vi "STA - Wave V2 Host.vi"() -> ()   [LabVIEW 2015]
doc: "The continuous acquisition mode tells the FPGA to acquire points indefinitely until a stop command is issued or until an error is encountered (FIFO overflow, module underflow, and so on). \n\nIn this acquisition mode, explicitly call the appropriate rwfm_ConfigTiming VI and set the host application's data buffer to be many times larger than the read size. The examples use a 10X size by default. If the host application's data buffer fills, then the FPGA experiences a FIFO overflow causing the acquisition to stop."
uses:
  <vilib>/rvi/interface/nirviOpenFPGA/nirviOpenFPGA.xnode
  <vilib>/rvi/interface/nirviCloseFPGA/nirviCloseFPGA.xnode
  <vilib>/NI/cRIO Wfm/cRIO Wfm.lvlib
  FPGA Bitfiles/SARAcqMain_9074.lvbitx
  C:/Program Files (x86)/National Instruments/LabVIEW 2015/ProjectTemplates/Source/cRIOWfm/FPGA/[FPGA] SAR Acq Main.vi
  <vilib>/FPGAPlugInAG/Dynamic/niLvFpga_Close_Dynamic.vi
  FPGA Bitfiles/STA-WaveformV0_FPGATarget2_[FPGA]DeltaSigMa_17CDL+fh61Q.lvbitx
  FPGA/[FPGA] DeltaSig Main.vi
  <vilib>/FPGAPlugInAG/cRIO-9112/niLvFpga_Open_cRIO-9112.vi
  <vilib>/rvi/interface/common/dynamic/niFpgaDynamicAddResources.vi
  <vilib>/NI/cRIO Wfm/ChannelConfig.ctl
panel:
  out "Array":timestamp[](array[timestamp])
  out "file path":path
  in  "error in (no error)":errorcluster
  out "error out":errorcluster
  in  "Sample Rate":u32=51200
  in  "stop":bool
  out "Waveform Graph":waveform(sgl)[](graph)
  in  "Channel Info":T1=[{"Channel Name"="Mod1/ai0", "Sensitivity mV_EU"=1000.0, "EU"="V", "dB Ref EU"=1.0}, {"Channel Name"="Mod1/ai1", "Sensitivity mV_EU"=1000.0, "EU"="V", "dB Ref EU"=1.0}, {"Channel Name"="Mod1/ai2", "Sensitivity mV_EU"=1000.0, "EU"="V", "dB Ref EU"=1.0}, {"Channel Name"="Mod1/ai3", "Sensitivity mV_EU"=1000.0, "EU"="V", "dB Ref EU"=1.0}] caption="Channel Name      Scale [mV/EU]        EU           dB Ref [EU]" {"dB Ref EU" format="%#.2p"; "Sensitivity mV_EU" format="%.2f"}
  in  "Samps per Chan":i32=25600 caption="Samples per Channel"
  out "Buffer Backlog":dbl caption="RT Buffer Backlog [%]" format="%#.2g"
  # "Sampling Info"
  # "Channel Info"
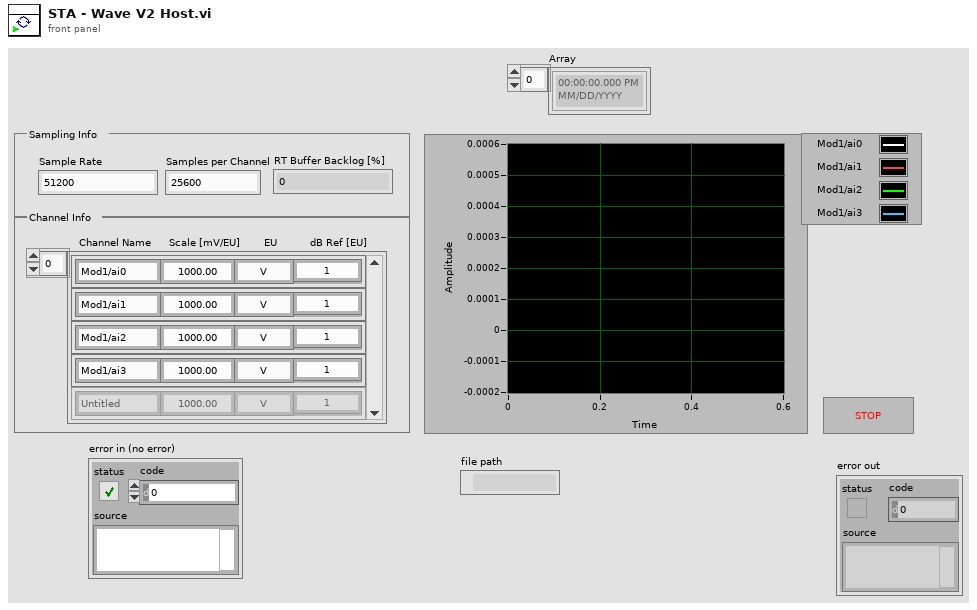
[diagram p1: front panel]
types:
  T1 = typedef "cRIO Wfm.lvlib/ChannelConfig.ctl" = cluster{"Channel Name":string, "Sensitivity mV_EU":dbl, "EU":string, "dB Ref EU":dbl}[]
  T2 = enum16{"open", "open or create", "create or replace", "create", "open (read-only)"}
  T3 = typedef "cRIO Wfm.lvlib/SamplingInfo.ctl" = cluster{"Number of Channels":i32, "Actual Samp Rate":dbl, "Chan Name Array":string[], "EU Chan Array":string[], "dB Ref Chan Array":dbl[]}
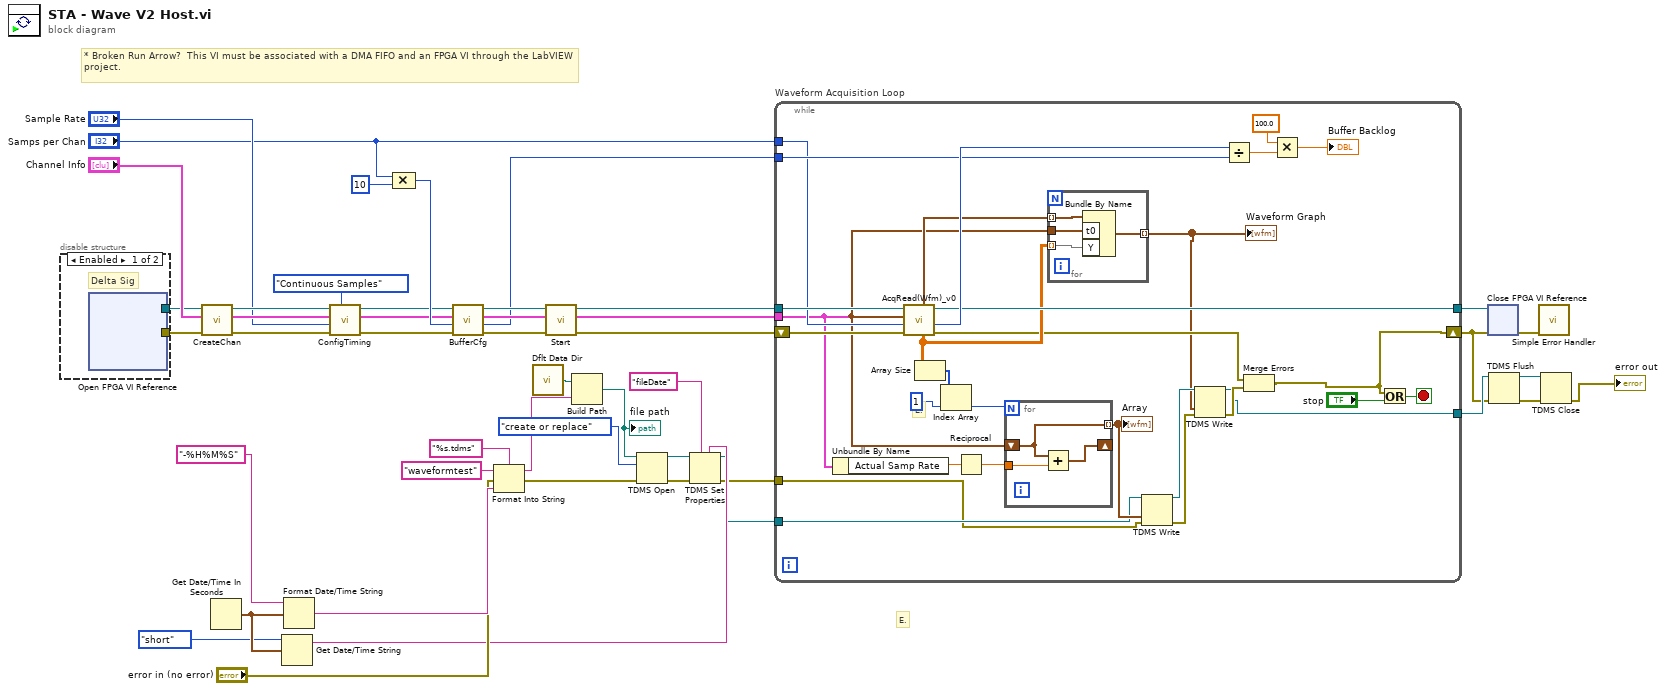
[diagram p0: block diagram]
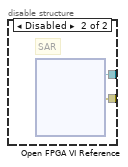
[diagram p2: hidden frame]
diagram:
  # "E."
  # "* Broken Run Arrow?  This VI must be associated with a DMA FIFO and an FPGA VI through the LabVIEW project."
  n1 = disable-structure shown="Enabled" {
    disable-tunnel: [w48 w50] -> w25
    disable-tunnel: [w47 w49] -> w24
    frame Enabled {
      # "Delta Sig"
      n2 = xnode "Open FPGA VI Reference"() -> ("FPGA VI Reference Out"=w48:refnum<k20>, "error out"=w47:errorcluster)  [unwired: 2 in]
    }
    frame Disabled {
      # "SAR"
      n3 = xnode "Open FPGA VI Reference"() -> ("FPGA VI Reference Out"=w50:refnum<k20>, "error out"=w49:errorcluster)  [unwired: 2 in]
    }
  }
  n4 = call <vilib>:"CreateChan.vi"("error in"=w24, "Channel Info"="Channel Info", "Dynamic FPGA Ref"=w25) -> ("error out"=w29:errorcluster, "Sampling Info"=w33:T3, "Dynamic FPGA Ref Out"=w34:refnum<k20>)  [unwired: 1 in, 5 out]
  n5 = Get Date/Time In Seconds() -> (seconds since 1Jan1904=w17:timestamp)
  n6 = Get Date/Time String(date format (0)=enum16{"short", "long", "abbreviated"}."short", seconds (now)=w17) -> (date string=w8:string)  [unwired: 1 in, 1 out]
  n7 = Format Date/Time String(time format string (%c)="-%H%M%S", seconds (now)=w17) -> (date/time string=w19:string)  [unwired: 1 in]
  n8 = call <vilib>:"ConfigTiming.vi"("Sample Mode"=enum16{"Finite Samples", "Continuous Samples"}."Continuous Samples", "error in"=w29, "Sample Rate"="Sample Rate", "Sampling Info In"=w33, "Dynamic FPGA Ref"=w34) -> ("error out"=w30:errorcluster, "Sampling Info Out"=w31:T3, "Dynamic FPGA Ref Out"=w32:refnum<k20>)  [unwired: 3 in, 1 out]
  n9 = Compound Arithmetic op=MULTIPLY("Samps per Chan", 10 ("value")) -> (w39:i32)
  n10 = call <vilib>:"BufferCfg.vi"("error in"=w30, "Buffer Size [Samps per Chan]"=w39, "Sampling Info In"=w31, "Dynamic FPGA Ref"=w32) -> ("error out"=w40:errorcluster, "Buffer Size [Total Samples]"=w36:u32, "Sampling Info Out"=w38:T3, "Dynamic FPGA Ref Out"=w41:refnum<k20>)  [unwired: 4 out]
  n11 = Format Into String(format string="%s.tdms", initial string="waveformtest", error in="error in (no error)", w19) -> (resulting string=w23:string, error out=w6:errorcluster)
  n12 = call <vilib>:"Dflt Data Dir.vi"() -> ("App:Default Data Directory"=w15:path)
  n13 = call <vilib>:"Start.vi"("error in"=w40, "Sampling Info In"=w38, "Dynamic FPGA Ref"=w41) -> ("error out"=w45:errorcluster, "Sampling Info Out"=w37:T3, "Dynamic FPGA Ref Out"=w46:refnum<k20>)  [unwired: 6 out]
  n14 = Build Path(base path=w15, name or relative path=w23) -> (appended path=w11:path)
  "file path" <- w11
  n15 = TDMS Open(8:w6, 10:T2."create or replace" ("operation (0:open)"), 11:w11) -> (0:w14:errorcluster, 3:w13:refnum<k34>)  [unwired: 4 in]
  n16 = TDMS Set Properties(5:w8, 7:"fileDate" ("property names"), 8:w14, 11:w13) -> (0:w4:errorcluster, 3:w5:refnum<k34>)  [unwired: 2 in, 2 out]
  n17 = while "Waveform Acquisition Loop" {
    tunnel: w46 -> [w74]
    tunnel: [w70] -> w44
    tunnel: w37 -> [w66]
    tunnel: w36 -> [w78]
    tunnel: "Samps per Chan" -> [w71]
    shift-right: [w62] -> w2
    shift-left: w45 -> [w80]
    tunnel: w5 -> [w60]
    tunnel: w4 -> [w59]
    tunnel: [w54] -> w3
    stop <- w73 stop-if-true
    # "E."
    n18 = Unbundle By Name(w66) -> ("Actual Samp Rate"=w65:dbl)
    n19 = call <vilib>:"AcqRead(Wfm)_v0.vi"("error in"=w80, "Samps Read per Chan"=w71, "Sampling Info"=w66, "Dynamic FPGA Ref"=w74) -> ("error out"=w63:errorcluster, "Samples Remaining"=w79:u32, "time stamp"=w67:timestamp, "Dynamic FPGA Ref Out"=w70:refnum<k20>, "transposed array"=w68:sgl[][], "Array"=w69:waveform(sgl)[])  [unwired: 2 in]
    n20 = Array Size(array=w68) -> (size(s)=w53:i32[])
    n21 = Index Array(array=w53, index=1) -> (element=w51:i32)
    n22 = Reciprocal(x=w65) -> (1/x=w64:dbl)
    n23 = for {
      N: w51 -> [_]
      shift-right: [w83] -> _
      shift-left: w67 -> [w82]
      tunnel: [w82] -> w61 mode=indexing
      tunnel: w64 -> [w81]
      n24 = Add(x=w82, y=w81) -> (x+y=w83:timestamp)
    }
    "Array" <- w61
    n25 = for {
      tunnel: w69 -> [w87] mode=indexing
      tunnel: w67 -> [w86]
      tunnel: [w85] -> w56 mode=indexing
      tunnel: w68 -> [w84] mode=indexing
      n26 = Bundle By Name(cluster=w87, "t0"=w86, "Y"=w84) -> (w85:waveform(sgl))
    }
    "Waveform Graph" <- w56
    n27 = TDMS Write(0:w60, 9:w61, 11:w59) -> (4:w57:refnum<k34>, 15:w58:errorcluster)  [unwired: 3 in, 2 out]
    n28 = TDMS Write(0:w57, 9:w56, 11:w58) -> (4:w54:refnum<k34>, 15:w55:errorcluster)  [unwired: 3 in, 2 out]
    n29 = Divide(x=w79, y=w78) -> (x/y=w77:dbl)
    n30 = Merge Errors(w63, w55) -> (w62:errorcluster)
    n31 = Multiply(x=100.0, y=w77) -> (x*y=→"Buffer Backlog":dbl)
    n32 = Or(x=w62, y="stop") -> (x .or. y?=w73:bool)
  }
  n33 = xnode "Close FPGA VI Reference"("FPGA VI Reference In"=w44, "error in"=w2) -> ("error out"=w42:errorcluster)
  n34 = TDMS Flush(4:w2, 7:w3) -> (0:w12:errorcluster, 3:w1:refnum<k34>)
  n35 = call <vilib>:"Simple Error Handler.vi"("error in (no error)"=w42) -> ()  [unwired: 1 in, 8 out]
  n36 = TDMS Close(8:w12, 11:w1) -> (0:→"error out":errorcluster)  [unwired: 1 out]
